vi "Boolean Array to SSD.vi"(7 "7 Segment Bool Array In":bool[](array[boolean])) -> (8 "7 Segment Out":string)   [LabVIEW 2016, in "2015 VA Washer.lvlib"]
uses:
  Projects/2015 VA Washer.lvlib
panel:
  # "A"
  # "B"
  # "C"
  # "D"
  # "E"
  # "F"
  # "G"
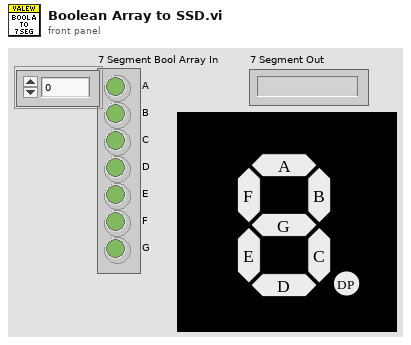
[diagram p1: front panel]
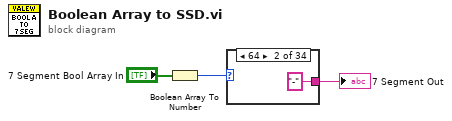
[diagram p0: block diagram]
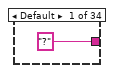
[diagram p2: hidden frame]
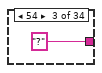
[diagram p3: hidden frame]
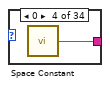
[diagram p4: hidden frame]
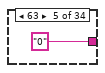
[diagram p5: hidden frame]
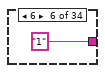
[diagram p6: hidden frame]
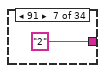
[diagram p7: hidden frame]
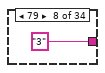
[diagram p8: hidden frame]
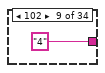
[diagram p9: hidden frame]
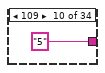
[diagram p10: hidden frame]
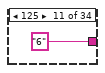
[diagram p11: hidden frame]
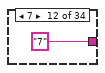
[diagram p12: hidden frame]
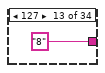
[diagram p13: hidden frame]
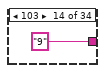
[diagram p14: hidden frame]
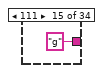
[diagram p15: hidden frame]
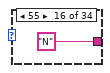
[diagram p16: hidden frame]
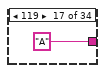
[diagram p17: hidden frame]
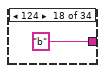
[diagram p18: hidden frame]
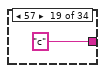
[diagram p19: hidden frame]
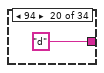
[diagram p20: hidden frame]
diagram:
  n1 = Boolean Array To Number(Boolean array="7 Segment Bool Array In") -> (number=w2:u32)
  n2 = case shown="64" w2 {
    tunnel: ["?" ("String") "-" ("String") "?" ("String") w7 "0" "1" "2" "3" "4" "5" "6" "7" "8" "9" "g" ("String") "N" ("String") "A" "b" "c" "d" ("String") "E" "F" "H" "I" "i" ("String") "J" "L" "n" "o" "P" "r" "T" "U" "Y"] -> w1
    frame Default {
    }
    frame 64 {
    }
    frame 54 {
    }
    frame 0 {
      n3 = call <vilib>:"Space Constant.vi"() -> ("String"=w7:string)
    }
    frame 63 {
    }
    frame 6 {
    }
    frame 91 {
    }
    frame 79 {
    }
    frame 102 {
    }
    frame 109 {
    }
    frame 125 {
    }
    frame 7 {
    }
    frame 127 {
    }
    frame 103 {
    }
    frame 111 {
    }
    frame 55 {
    }
    frame 119 {
    }
    frame 124 {
    }
    frame 57 {
    }
    frame 94 {
    }
    frame 121 {
    }
    frame 113 {
    }
    frame 118 {
    }
    frame 48 {
    }
    frame 16 {
    }
    frame 15 {
    }
    frame 56 {
    }
    frame 84 {
    }
    frame 92 {
    }
    frame 115 {
    }
    frame 80 {
    }
    frame 120 {
    }
    frame 62 {
    }
    frame 110 {
    }
  }
  "7 Segment Out" <- w1
